vi "USB RAW - Bulk.vi"() -> ()   [LabVIEW 2023]
doc: "This example shows how to read and write simple user events from and to a USB RAW device. \n\n<b>Note:</b> This example works only with USB RAW devices.\n\nBefore you run this VI, install a USB RAW device and configure NI Measurement & Automation Explorer (MAX) to recognize the USB device. You can read to and write from the USB RAW device only after you install and configure the USB RAW device and open a session to the device. To read to or write from another device, close the session to the current device, select another device from the <b>VISA Resource</b> control, and open a session to the new device. \n\nWhen you complete the read or write, click the <b>Stop</b> button to stop the VI."
panel:
  in  "Not USB":string="The specified VISA resource is not a USB device."
  out "Bulk Read Response":string
  in  "Stop":bool
  in  "VISA Resource":refnum<visa-resource-name>
  in  "Bulk Write Data":string="*IDN?\n"
  in  "Bulk In":bool
  in  "Bulk Out":bool
  # "Overview: Demonstrates the use of the VISA functions to communicate to a USB RAW device.\nRequirements: NI-VISA Driver, USB RAW device\nInstructions:\n1. Ensure the USB RAW device specified by the VISA Resource control is properly configured in Measurement & Automation Explorer.\n2. Run the VI.\n3. Click the Bulk Out and Bulk In buttons to write to/read from your USB RAW device.\n4. Click Stop to stop the VI."
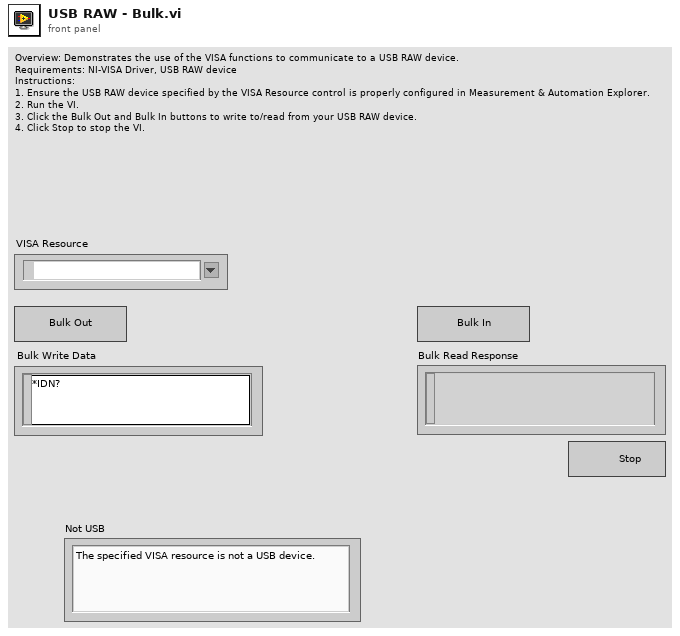
[diagram p1: front panel]
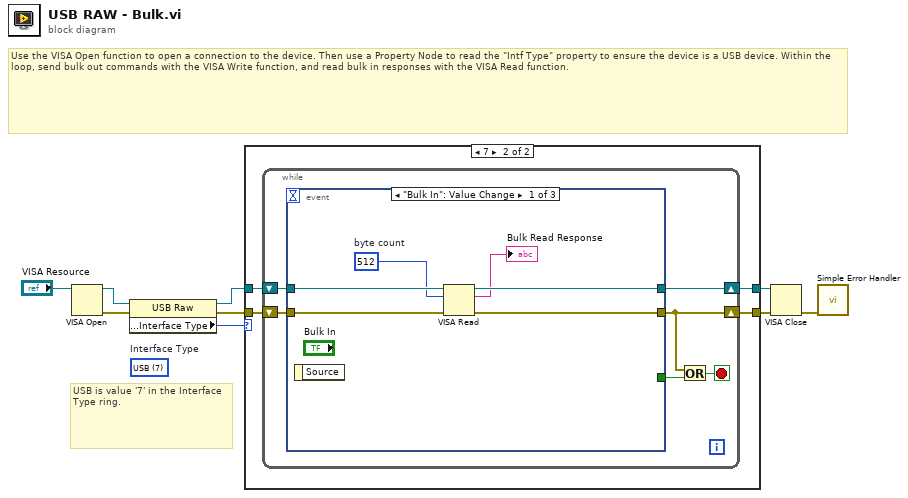
[diagram p0: block diagram]
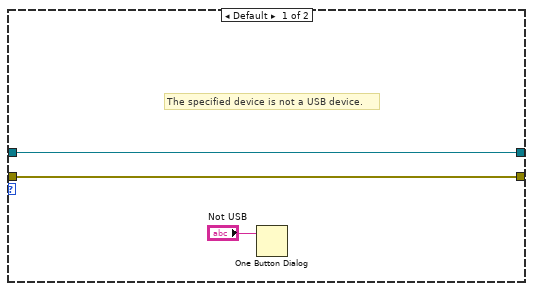
[diagram p2: hidden frame]
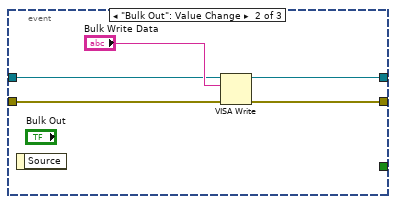
[diagram p3: hidden frame]
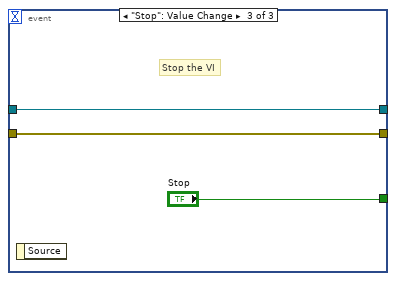
[diagram p4: hidden frame]
diagram:
  (unwired) u16 7 items=["GPIB"=1, "VXI"=2, "GPIB-VXI"=3, "Serial"=4, "PXI"=5, "TCPIP"=6, "USB"=7, "FireWire"=9]  # Interface Type
  # "Use the VISA Open function to open a connection to the device. Then use a Property Node to read the \"Intf Type\" property to ensure the device is a USB device. Within the loop, send bulk out commands with the VISA Write function, and read bulk in responses with the VISA Read function."
  # "USB is value '7' in the Interface Type ring."
  n1 = VISA Open(VISA resource name="VISA Resource") -> (VISA resource name=w8:refnum<visa-resource-name>, error out=w9:errorcluster)  [unwired: 1 in, 3 out]
  n2 = property class="USB Raw"(reference=w8, error in=w9) -> (reference out=w2:refnum<visa-resource-name>, error out=w3:errorcluster, "Interface Information:Interface Type"=w1:u16)
  n3 = case shown="7" w1 {
    tunnel: [w12 w16] -> w6
    tunnel: [w11 w15] -> w4
    tunnel: w3 -> [w12 w14]
    tunnel: w2 -> [w11 w13]
    frame Default {
      # "The specified device is not a USB device."
      n4 = One Button Dialog(message="Not USB") -> ()  [unwired: 1 in, 1 out]
    }
    frame 7 {
      n5 = while {
        shift-right: [w18] -> w16
        shift-left: w14 -> [w17]
        shift-right: [w20] -> w15
        shift-left: w13 -> [w19]
        stop <- w21 stop-if-true
        n6 = event shown="[0] \"Bulk In\": Value Change" {
          selector: _ -> [_ _ _]
          dyn-events: _ -> [_ _ _]
          timeout: _ -> [_ _ _]
          tunnel: [_ _ "Stop"] -> w22
          tunnel: [w28 w32 w34] -> w18
          tunnel: w17 -> [w26 w33 w34]
          tunnel: [w27 w31 w35] -> w20
          tunnel: w19 -> [w25 w29 w35]
          event "Bulk In": Value Change {
            w24 = u32 512  # byte count
            n7 = event-data() -> ()  [unwired: 2 out]
            n8 = VISA Read(VISA resource name=w25, byte count=w24, error in (no error)=w26) -> (VISA resource name out=w27:refnum<visa-resource-name>, read buffer=→"Bulk Read Response":string, error out=w28:errorcluster)  [unwired: 1 out]
          }
          event "Bulk Out": Value Change {
            n9 = event-data() -> ()  [unwired: 2 out]
            n10 = VISA Write(VISA resource name=w29, write buffer="Bulk Write Data", error in (no error)=w33) -> (VISA resource name out=w31:refnum<visa-resource-name>, error out=w32:errorcluster)  [unwired: 1 out]
          }
          event "Stop": Value Change {
            # "Stop the VI"
            n11 = event-data() -> ()  [unwired: 2 out]
          }
        }
        n12 = Or(x=w18, y=w22) -> (x .or. y?=w21:bool)
      }
    }
  }
  n13 = VISA Close(VISA resource name=w4, error in (no error)=w6) -> (error out=w5:errorcluster)
  n14 = call <vilib>:"Simple Error Handler.vi"("error in (no error)"=w5) -> ()  [unwired: 1 in, 8 out]
